vi "Execute Command.vi"(6 "Gantry In":refnum<class "Gantry.lvclass">, 7 "Console Log In":refnum<class "Console Log.lvclass">, 8 "error in (no error)":errorcluster, 9 "Pause in":bool, 10 "Command":string, 11 "gScript Interpreter in":refnum<class "gScript Interpreter.lvclass">) -> (0 "error out":errorcluster, 1 "Pause out":bool, 2 "End out":bool, 3 "gScript Interpreter out":refnum<class "gScript Interpreter.lvclass">, 4 "Gantry Out":refnum<class "Gantry.lvclass">, 5 "Console Log Out":refnum<class "Console Log.lvclass">)   [LabVIEW 2017, in "gScript Interpreter.lvclass"]
uses:
  gScript Interpreter.lvclass
  Shared Components/Gantry Class/Gantry.lvclass
  Application Utilities/Console Log/Console Log.lvclass
  gScript Interpreter.lvclass/gScript Interpreter.ctl
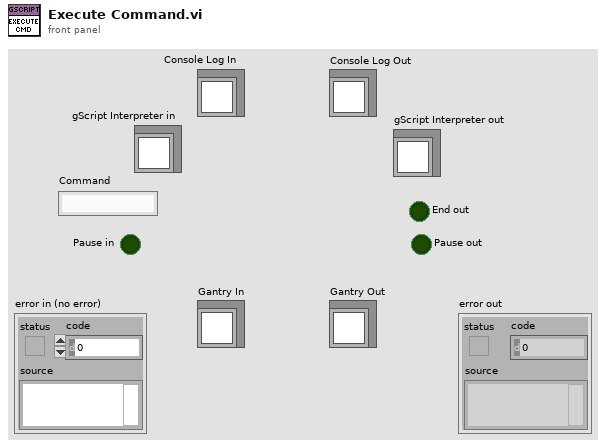
[diagram p1: front panel]
types:
  T1 = typedef "Command.ctl" = enum16{"", "PASS", "COPY", "PRINT", "GOTO", "GOTOIF", "GOTOIFN", "ADD", "SUB", "INC", "DEC", "HOME", "MOVEREL", "MOVENAME", "MOVETO", "GETPOS", "ROTATE", "GETROT", "SETVAC", "GETVAC", "JOYSTICK", "LOADTOOL", "UNLOADTOOL", "POTLINE", "POTDOT", "AUTOFOCUS", "FINDFID", "FIT", "WAIT", "MPGON", "MPGOFF", "PAUSE", "SNAPSHOT", "SETLOG", "CLEARLOG", "VIDEO", "TRANSFORMG2L", "TRANSFORML2G", "CHOICEPOPUP", "SETLIGHT", "CALL", "END", "DUMPSTATE", "FLEXREAD", "FLEXWRITE", "SURVEY", "LOADCONFIG", "SETERRORMODE", "COMPOSE", "INVERT", "EULER2QUAT", "QUAT2EULER", "MUL", "ROTATETO", "VERSION", "SIN", "COS", "TAN", "ATAN2", "ABS", "POW", "ACKFAULT", "MOVESAFE", "LOADSTAMP", "APPLYSTAMP", "UNLOADSTAMP", "LOADWEIGHT", "APPLYWEIGHT", "UNLOADWEIGHT", "RETURN", "GETFLOATPOPUP", "GETINTPOPUP", "GETVECPOPUP"}
  T2 = typedef "Error Mode.ctl" = enum16{"default", "prompt", "setvar"}
  T3 = typedef "Memory Cell.ctl" = cluster{"type":T4, "x":dbl, "y":dbl, "z":dbl, "w":dbl}
  T4 = typedef "Memory Cell Type Enum.ctl" = enum16{"integer", "float", "vector", "rotation"}
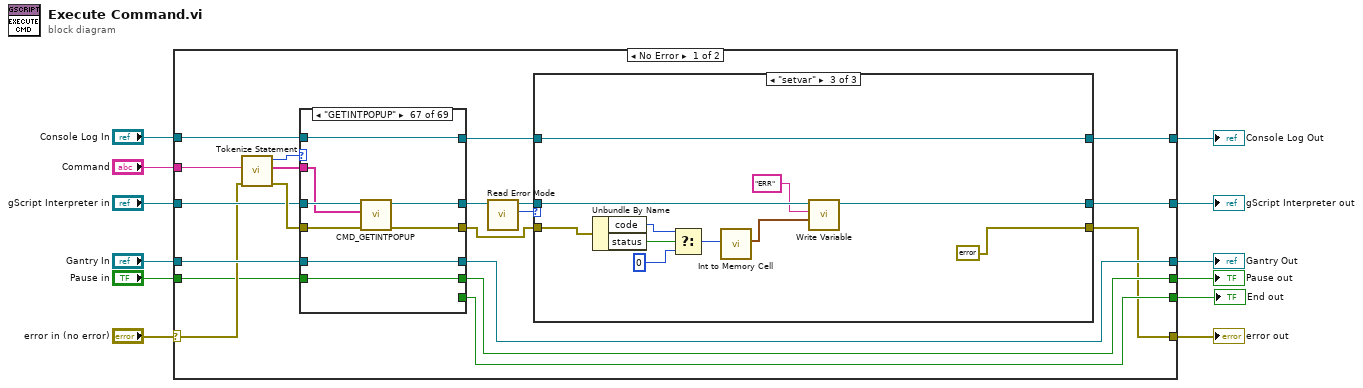
[diagram p0: block diagram]
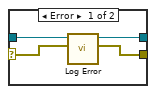
[diagram p3: hidden frame]
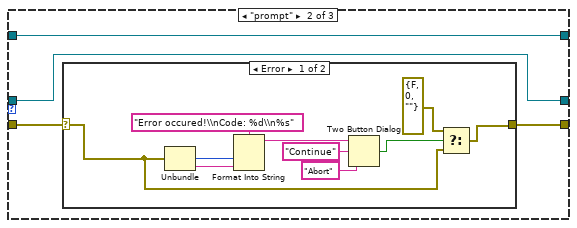
[diagram p4: hidden frame]
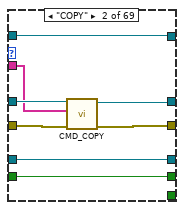
[diagram p7: hidden frame]
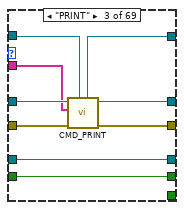
[diagram p8: hidden frame]
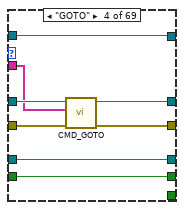
[diagram p9: hidden frame]
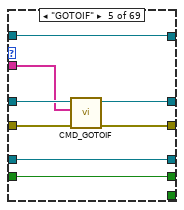
[diagram p10: hidden frame]
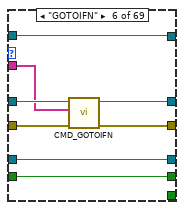
[diagram p11: hidden frame]
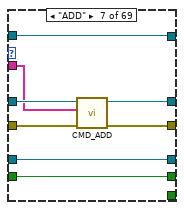
[diagram p12: hidden frame]
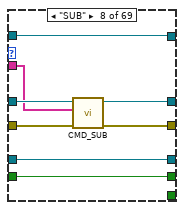
[diagram p13: hidden frame]
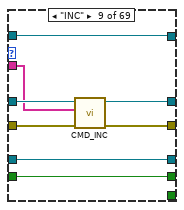
[diagram p14: hidden frame]
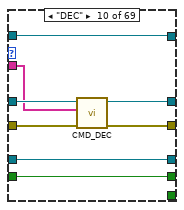
[diagram p15: hidden frame]
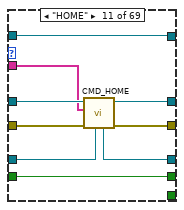
[diagram p16: hidden frame]
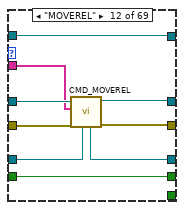
[diagram p17: hidden frame]
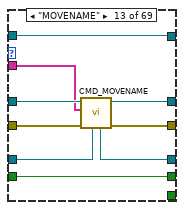
[diagram p18: hidden frame]
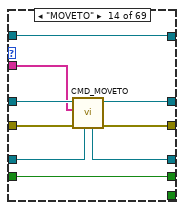
[diagram p19: hidden frame]
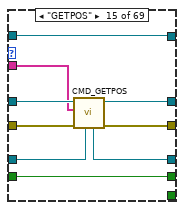
[diagram p20: hidden frame]
diagram:
  n1 = case shown="No Error" "error in (no error)" {
    selector: "error in (no error)" -> [w26 w662]
    tunnel: [w19 w662] -> w11
    tunnel: [w18 w661] -> w9
    tunnel: "gScript Interpreter in" -> [w28 w661]
    tunnel: "Gantry In" -> [w29 w659]
    tunnel: [w21 w659] -> w7
    tunnel: "Console Log In" -> [w27 w660]
    tunnel: [w16 w660] -> w5
    tunnel: "Pause in" -> [w25 w658]
    tunnel: [w22 w658] -> w3
    tunnel: "Command" -> [w24 _]
    tunnel: [w23 FALSE] -> w1
    frame No Error {
      n2 = call "Tokenize Statement.vi"("error in (no error)"=w26, "Command"=w24) -> ("error out"=w30:errorcluster, "Arguments"=w31:string[], "Command"=w32:T1)  [unwired: 5 in, 2 out]
      n3 = case shown="\"GETINTPOPUP\"" w32 {
        selector: w32 -> [_ _ _ _ _ _ _ _ _ _ _ _ _ _ _ _ _ _ _ _ _ _ _ _ _ _ _ _ _ _ _ _ _ _ _ _ _ _ _ _ _ _ _ _ _ _ _ _ _ _ _ _ _ _ _ _ _ _ _ _ _ w586 _ w605 w615 _ _ _ _]
        tunnel: w31 -> [_ w78 w87 w95 w102 w110 w118 w127 w135 w142 w150 w159 w172 w179 w186 w195 w204 w213 w222 w231 w244 w249 w263 w267 w276 w285 w294 w306 w311 w320 _ w339 w345 w351 w370 w376 w381 w389 w401 w409 _ w418 w429 w441 w453 w455 w464 w472 w480 w491 w499 w509 w512 w521 w529 w539 w545 w553 w564 w569 w581 w593 w596 w606 w617 w625 w633 w642 w649]
        tunnel: w30 -> [w72 w80 w89 w97 w104 w113 w121 w129 w137 w144 w155 w163 w171 w181 w190 w199 w208 w216 w224 w235 w243 w251 w262 w271 w280 w287 w298 w305 w313 w324 w330 w335 w344 w354 w365 w374 w380 w390 w400 w405 w412 w422 w433 w442 w447 w459 w466 w477 w484 w492 w500 w506 w518 w524 w534 w541 w548 w556 w565 w572 w580 w590 w600 w608 w621 w629 w636 w645 w652]
        tunnel: w28 -> [w74 w82 w91 w99 w107 w115 w123 w131 w139 w146 w156 w165 w174 w183 w192 w201 w210 w219 w228 w237 w246 w255 w264 w273 w282 w291 w300 w308 w317 w326 w331 w338 w347 w356 w369 w377 w385 w393 w402 w408 w415 w420 w435 w444 w452 w461 w468 w476 w486 w493 w502 w508 w519 w526 w535 w543 w551 w559 w567 w575 w583 w592 w599 w612 w623 w628 w639 w646 w654]
        tunnel: [w74 w81 w90 w98 w106 w114 w122 w130 w138 w145 w151 w164 w173 w182 w191 w200 w209 w214 w227 w236 w245 w254 w260 w272 w281 w290 w299 w307 w316 w325 w331 w337 w346 w355 w368 w375 w382 w392 w399 w407 w415 w419 w434 w443 w451 w460 w467 w475 w485 w490 w501 w507 w514 w525 w532 w542 w550 w558 w566 w574 w582 w591 w598 w611 w622 w627 w637 w641 w653] -> w20
        tunnel: [w72 w79 w88 w96 w103 w112 w120 w128 w136 w143 w154 w162 w168 w180 w189 w198 w207 w215 w223 w234 w242 w250 w261 w270 w279 w286 w297 w304 w312 w323 w330 w334 w343 w353 w364 w372 w379 w388 w398 w404 w412 w421 w432 w440 w446 w458 w465 w474 w483 w489 w498 w505 w515 w523 w533 w540 w547 w555 w563 w571 w579 w589 w597 w607 w620 w626 w634 w644 w651] -> w15
        tunnel: w29 -> [w73 w77 w86 w94 w105 w111 w119 w126 w134 w147 w153 w161 w170 w178 w188 w197 w206 w218 w226 w233 w241 w253 w259 w269 w278 w289 w296 w303 w315 w322 w329 w333 w342 w352 w367 w373 w384 w387 w397 w406 w414 w424 w431 w439 w449 w457 w469 w478 w482 w488 w497 w504 w517 w522 w530 w537 w546 w554 w561 w570 w578 w588 w602 w610 w619 w630 w635 w643 w650]
        tunnel: [w73 w77 w86 w94 w105 w111 w119 w126 w134 w147 w152 w160 w169 w177 w187 w196 w205 w217 w225 w232 w240 w252 w258 w268 w277 w288 w295 w303 w314 w321 w329 w332 w341 w352 w366 w373 w384 w387 w396 w406 w414 w423 w430 w438 w448 w456 w469 w478 w482 w488 w497 w504 w516 w522 w530 w537 w546 w554 w561 w570 w577 w587 w601 w609 w618 w630 w635 w643 w650] -> w21
        tunnel: w25 -> [w71 w76 w85 w93 w101 w109 w117 w125 w133 w141 w149 w158 w167 w176 w185 w194 w203 w212 w221 w230 w239 w248 w257 w266 w275 w284 w293 w302 w310 w319 _ w340 w350 w359 w362 w378 w386 w394 w403 w411 w417 w427 w436 w445 w454 w463 w471 w479 w487 w495 w503 w511 w520 w528 w536 w544 w552 w560 w568 w576 w585 w595 w604 w614 w624 w632 w640 w648 w656]
        tunnel: [w71 w76 w85 w93 w101 w109 w117 w125 w133 w141 w149 w158 w167 w176 w185 w194 w203 w212 w221 w230 w239 w248 w257 w266 w275 w284 w293 w302 w310 w319 TRUE w340 w350 w359 w360 w378 w386 w394 w403 w411 w417 w427 w436 w445 w454 w463 w471 w479 w487 w495 w503 w511 w520 w528 w536 w544 w552 w560 w568 w576 w585 w595 w604 w614 w624 w632 w640 w648 w656] -> w22
        tunnel: w27 -> [w70 w75 w84 w92 w100 w108 w116 w124 w132 w140 w148 w157 w166 w175 w184 w193 w202 w211 w220 w229 w238 w247 w256 w265 w274 w283 w292 w301 w309 w318 w327 w336 w349 w358 w363 w371 w383 w391 w395 w410 w416 w426 w428 w437 w450 w462 w470 w473 w481 w494 w496 w510 w513 w527 w531 w538 w549 w557 w562 w573 w584 w594 w603 w613 w616 w631 w638 w647 w655]
        tunnel: [w70 w75 w83 w92 w100 w108 w116 w124 w132 w140 w148 w157 w166 w175 w184 w193 w202 w211 w220 w229 w238 w247 w256 w265 w274 w283 w292 w301 w309 w318 w327 w336 w348 w357 w363 w371 w383 w391 w395 w410 w416 w425 w428 w437 w450 w462 w470 w473 w481 w494 w496 w510 w513 w527 w531 w538 w549 w557 w562 w573 w584 w594 w603 w613 w616 w631 w638 w647 w655] -> w17
        tunnel: [_ _ _ _ _ _ _ _ _ _ _ _ _ _ _ _ _ _ _ _ _ _ _ _ _ _ _ _ _ _ _ _ _ _ _ _ _ _ _ _ TRUE _ _ _ _ _ _ _ _ _ _ _ _ _ _ _ _ _ _ _ _ _ _ _ _ _ _ _ _] -> w23
        frame "PASS", Default {
        }
        frame "COPY" {
          n4 = call-dynamic "CMD_COPY.vi"("error in (no error)"=w80, "Arguments"=w78, "gScript Interpreter in"=w82) -> ("error out"=w79:errorcluster, "gScript Interpreter out"=w81:refnum<class "gScript Interpreter.lvclass">)  [unwired: 7 in]
        }
        frame "PRINT" {
          n5 = call-dynamic "CMD_PRINT.vi"("Console Log in"=w84, "error in (no error)"=w89, "Arguments"=w87, "gScript Interpreter in"=w91) -> ("error out"=w88:errorcluster, "gScript Interpreter out"=w90:refnum<class "gScript Interpreter.lvclass">, "Console Log out"=w83:refnum<class "Console Log.lvclass">)  [unwired: 5 in]
        }
        frame "GOTO" {
          n6 = call-dynamic "CMD_GOTO.vi"("error in (no error)"=w97, "Arguments"=w95, "gScript Interpreter in"=w99) -> ("error out"=w96:errorcluster, "gScript Interpreter out"=w98:refnum<class "gScript Interpreter.lvclass">)  [unwired: 7 in]
        }
        frame "GOTOIF" {
          n7 = call-dynamic "CMD_GOTOIF.vi"("error in (no error)"=w104, "Arguments"=w102, "gScript Interpreter in"=w107) -> ("error out"=w103:errorcluster, "gScript Interpreter out"=w106:refnum<class "gScript Interpreter.lvclass">)  [unwired: 7 in]
        }
        frame "GOTOIFN" {
          n8 = call-dynamic "CMD_GOTOIFN.vi"("error in (no error)"=w113, "Arguments"=w110, "gScript Interpreter in"=w115) -> ("error out"=w112:errorcluster, "gScript Interpreter out"=w114:refnum<class "gScript Interpreter.lvclass">)  [unwired: 7 in]
        }
        frame "ADD" {
          n9 = call-dynamic "CMD_ADD.vi"("error in (no error)"=w121, "Arguments"=w118, "gScript Interpreter in"=w123) -> ("error out"=w120:errorcluster, "gScript Interpreter out"=w122:refnum<class "gScript Interpreter.lvclass">)  [unwired: 7 in]
        }
        frame "SUB" {
          n10 = call-dynamic "CMD_SUB.vi"("error in (no error)"=w129, "Arguments"=w127, "gScript Interpreter in"=w131) -> ("error out"=w128:errorcluster, "gScript Interpreter out"=w130:refnum<class "gScript Interpreter.lvclass">)  [unwired: 7 in]
        }
        frame "INC" {
          n11 = call-dynamic "CMD_INC.vi"("error in (no error)"=w137, "Arguments"=w135, "gScript Interpreter in"=w139) -> ("error out"=w136:errorcluster, "gScript Interpreter out"=w138:refnum<class "gScript Interpreter.lvclass">)  [unwired: 7 in]
        }
        frame "DEC" {
          n12 = call-dynamic "CMD_DEC.vi"("error in (no error)"=w144, "Arguments"=w142, "gScript Interpreter in"=w146) -> ("error out"=w143:errorcluster, "gScript Interpreter out"=w145:refnum<class "gScript Interpreter.lvclass">)  [unwired: 7 in]
        }
        frame "HOME" {
          n13 = call-dynamic "CMD_HOME.vi"("Gantry in"=w153, "error in (no error)"=w155, "Arguments"=w150, "gScript Interpreter in"=w156) -> ("error out"=w154:errorcluster, "gScript Interpreter out"=w151:refnum<class "gScript Interpreter.lvclass">, "Gantry out"=w152:refnum<class "Gantry.lvclass">)  [unwired: 5 in]
        }
        frame "MOVEREL" {
          n14 = call-dynamic "CMD_MOVEREL.vi"("Gantry in"=w161, "error in (no error)"=w163, "Arguments"=w159, "gScript Interpreter in"=w165) -> ("error out"=w162:errorcluster, "gScript Interpreter out"=w164:refnum<class "gScript Interpreter.lvclass">, "Gantry out"=w160:refnum<class "Gantry.lvclass">)  [unwired: 5 in]
        }
        frame "MOVENAME" {
          n15 = call-dynamic "CMD_MOVENAME.vi"("Gantry in"=w170, "error in (no error)"=w171, "Arguments"=w172, "gScript Interpreter in"=w174) -> ("error out"=w168:errorcluster, "gScript Interpreter out"=w173:refnum<class "gScript Interpreter.lvclass">, "Gantry out"=w169:refnum<class "Gantry.lvclass">)  [unwired: 5 in]
        }
        frame "MOVETO" {
          n16 = call-dynamic "CMD_MOVETO.vi"("Gantry in"=w178, "error in (no error)"=w181, "Arguments"=w179, "gScript Interpreter in"=w183) -> ("error out"=w180:errorcluster, "gScript Interpreter out"=w182:refnum<class "gScript Interpreter.lvclass">, "Gantry out"=w177:refnum<class "Gantry.lvclass">)  [unwired: 5 in]
        }
        frame "GETPOS" {
          n17 = call-dynamic "CMD_GETPOS.vi"("Gantry in"=w188, "error in (no error)"=w190, "Arguments"=w186, "gScript Interpreter in"=w192) -> ("error out"=w189:errorcluster, "gScript Interpreter out"=w191:refnum<class "gScript Interpreter.lvclass">, "Gantry out"=w187:refnum<class "Gantry.lvclass">)  [unwired: 5 in]
        }
        frame "ROTATE" {
          n18 = call-dynamic "CMD_ROTATE.vi"("Gantry in"=w197, "error in (no error)"=w199, "Arguments"=w195, "gScript Interpreter in"=w201) -> ("error out"=w198:errorcluster, "gScript Interpreter out"=w200:refnum<class "gScript Interpreter.lvclass">, "Gantry out"=w196:refnum<class "Gantry.lvclass">)  [unwired: 5 in]
        }
        frame "GETROT" {
          n19 = call-dynamic "CMD_GETROT.vi"("Gantry in"=w206, "error in (no error)"=w208, "Arguments"=w204, "gScript Interpreter in"=w210) -> ("error out"=w207:errorcluster, "gScript Interpreter out"=w209:refnum<class "gScript Interpreter.lvclass">, "Gantry out"=w205:refnum<class "Gantry.lvclass">)  [unwired: 5 in]
        }
        frame "SETVAC" {
          n20 = call-dynamic "CMD_SETVAC.vi"("Gantry in"=w218, "error in (no error)"=w216, "Arguments"=w213, "gScript Interpreter in"=w219) -> ("error out"=w215:errorcluster, "gScript Interpreter out"=w214:refnum<class "gScript Interpreter.lvclass">, "Gantry out"=w217:refnum<class "Gantry.lvclass">)  [unwired: 5 in]
        }
        frame "GETVAC" {
          n21 = call-dynamic "CMD_GETVAC.vi"("Gantry in"=w226, "error in (no error)"=w224, "Arguments"=w222, "gScript Interpreter in"=w228) -> ("error out"=w223:errorcluster, "gScript Interpreter out"=w227:refnum<class "gScript Interpreter.lvclass">, "Gantry out"=w225:refnum<class "Gantry.lvclass">)  [unwired: 5 in]
        }
        frame "JOYSTICK" {
          n22 = call-dynamic "CMD_JOYSTICK.vi"("Gantry in"=w233, "error in (no error)"=w235, "Arguments"=w231, "gScript Interpreter in"=w237) -> ("error out"=w234:errorcluster, "gScript Interpreter out"=w236:refnum<class "gScript Interpreter.lvclass">, "Gantry out"=w232:refnum<class "Gantry.lvclass">)  [unwired: 5 in]
        }
        frame "LOADTOOL" {
          n23 = call-dynamic "CMD_LOADTOOL.vi"("Gantry in"=w241, "error in (no error)"=w243, "Arguments"=w244, "gScript Interpreter in"=w246) -> ("error out"=w242:errorcluster, "gScript Interpreter out"=w245:refnum<class "gScript Interpreter.lvclass">, "Gantry out"=w240:refnum<class "Gantry.lvclass">)  [unwired: 5 in]
        }
        frame "UNLOADTOOL" {
          n24 = call-dynamic "CMD_UNLOADTOOL.vi"("Gantry in"=w253, "error in (no error)"=w251, "Arguments"=w249, "gScript Interpreter in"=w255) -> ("error out"=w250:errorcluster, "gScript Interpreter out"=w254:refnum<class "gScript Interpreter.lvclass">, "Gantry out"=w252:refnum<class "Gantry.lvclass">)  [unwired: 5 in]
        }
        frame "POTLINE" {
          n25 = call-dynamic "CMD_POTLINE.vi"("Gantry in"=w259, "error in (no error)"=w262, "Arguments"=w263, "gScript Interpreter in"=w264) -> ("error out"=w261:errorcluster, "gScript Interpreter out"=w260:refnum<class "gScript Interpreter.lvclass">, "Gantry out"=w258:refnum<class "Gantry.lvclass">)  [unwired: 5 in]
        }
        frame "POTDOT" {
          n26 = call-dynamic "CMD_POTDOT.vi"("Gantry in"=w269, "error in (no error)"=w271, "Arguments"=w267, "gScript Interpreter in"=w273) -> ("error out"=w270:errorcluster, "gScript Interpreter out"=w272:refnum<class "gScript Interpreter.lvclass">, "Gantry out"=w268:refnum<class "Gantry.lvclass">)  [unwired: 5 in]
        }
        frame "AUTOFOCUS" {
          n27 = call-dynamic "CMD_AUTOFOCUS.vi"("Gantry in"=w278, "error in (no error)"=w280, "Arguments"=w276, "gScript Interpreter in"=w282) -> ("error out"=w279:errorcluster, "gScript Interpreter out"=w281:refnum<class "gScript Interpreter.lvclass">, "Gantry out"=w277:refnum<class "Gantry.lvclass">)  [unwired: 5 in]
        }
        frame "FINDFID" {
          n28 = call-dynamic "CMD_FINDFID.vi"("Gantry in"=w289, "error in (no error)"=w287, "Arguments"=w285, "gScript Interpreter in"=w291) -> ("error out"=w286:errorcluster, "gScript Interpreter out"=w290:refnum<class "gScript Interpreter.lvclass">, "Gantry out"=w288:refnum<class "Gantry.lvclass">)  [unwired: 5 in]
        }
        frame "FIT" {
          n29 = call-dynamic "CMD_FIT.vi"("Gantry in"=w296, "error in (no error)"=w298, "Arguments"=w294, "gScript Interpreter in"=w300) -> ("error out"=w297:errorcluster, "gScript Interpreter out"=w299:refnum<class "gScript Interpreter.lvclass">, "Gantry out"=w295:refnum<class "Gantry.lvclass">)  [unwired: 5 in]
        }
        frame "WAIT" {
          n30 = call-dynamic "CMD_WAIT.vi"("error in (no error)"=w305, "Arguments"=w306, "gScript Interpreter in"=w308) -> ("error out"=w304:errorcluster, "gScript Interpreter out"=w307:refnum<class "gScript Interpreter.lvclass">)  [unwired: 7 in]
        }
        frame "MPGON" {
          n31 = call-dynamic "CMD_MPGON.vi"("Gantry in"=w315, "error in (no error)"=w313, "Arguments"=w311, "gScript Interpreter in"=w317) -> ("error out"=w312:errorcluster, "gScript Interpreter out"=w316:refnum<class "gScript Interpreter.lvclass">, "Gantry out"=w314:refnum<class "Gantry.lvclass">)  [unwired: 5 in]
        }
        frame "MPGOFF" {
          n32 = call-dynamic "CMD_MPGOFF.vi"("Gantry in"=w322, "error in (no error)"=w324, "Arguments"=w320, "gScript Interpreter in"=w326) -> ("error out"=w323:errorcluster, "gScript Interpreter out"=w325:refnum<class "gScript Interpreter.lvclass">, "Gantry out"=w321:refnum<class "Gantry.lvclass">)  [unwired: 5 in]
        }
        frame "PAUSE" {
        }
        frame "SNAPSHOT" {
          n33 = call-dynamic "CMD_SNAPSHOT.vi"("Gantry in"=w333, "error in (no error)"=w335, "Arguments"=w339, "gScript Interpreter in"=w338) -> ("error out"=w334:errorcluster, "gScript Interpreter out"=w337:refnum<class "gScript Interpreter.lvclass">, "Gantry out"=w332:refnum<class "Gantry.lvclass">)  [unwired: 5 in]
        }
        frame "SETLOG" {
          n34 = call-dynamic "CMD_SETLOG.vi"("Gantry Class in"=w342, "Console Log in"=w349, "error in (no error)"=w344, "Arguments"=w345, "gScript Interpreter in"=w347) -> ("error out"=w343:errorcluster, "gScript Interpreter out"=w346:refnum<class "gScript Interpreter.lvclass">, "Gantry Class out"=w341:refnum<class "Gantry.lvclass">, "Console Log out"=w348:refnum<class "Console Log.lvclass">)  [unwired: 3 in]
        }
        frame "CLEARLOG" {
          n35 = call-dynamic "CMD_CLEARLOG.vi"("Console Log in"=w358, "error in (no error)"=w354, "Arguments"=w351, "gScript Interpreter in"=w356) -> ("error out"=w353:errorcluster, "gScript Interpreter out"=w355:refnum<class "gScript Interpreter.lvclass">, "Console Log out"=w357:refnum<class "Console Log.lvclass">)  [unwired: 5 in]
        }
        frame "VIDEO" {
          n36 = call-dynamic "CMD_VIDEO.vi"("Gantry in"=w367, "error in (no error)"=w365, "Arguments"=w370, "gScript Interpreter in"=w369) -> ("error out"=w364:errorcluster, "Pause out"=w361:bool, "gScript Interpreter out"=w368:refnum<class "gScript Interpreter.lvclass">, "Gantry out"=w366:refnum<class "Gantry.lvclass">)  [unwired: 4 in]
          n37 = Or(x=w361, y=w362) -> (x .or. y?=w360:bool)
        }
        frame "TRANSFORMG2L" {
          n38 = call-dynamic "CMD_TRANSFORMG2L.vi"("error in (no error)"=w374, "Arguments"=w376, "gScript Interpreter in"=w377) -> ("error out"=w372:errorcluster, "gScript Interpreter out"=w375:refnum<class "gScript Interpreter.lvclass">)  [unwired: 7 in]
        }
        frame "TRANSFORML2G" {
          n39 = call-dynamic "CMD_TRANSFORML2G.vi"("error in (no error)"=w380, "Arguments"=w381, "gScript Interpreter in"=w385) -> ("error out"=w379:errorcluster, "gScript Interpreter out"=w382:refnum<class "gScript Interpreter.lvclass">)  [unwired: 7 in]
        }
        frame "CHOICEPOPUP" {
          n40 = call-dynamic "CMD_CHOICEPOPUP.vi"("error in (no error)"=w390, "Arguments"=w389, "gScript Interpreter in"=w393) -> ("error out"=w388:errorcluster, "gScript Interpreter out"=w392:refnum<class "gScript Interpreter.lvclass">)  [unwired: 7 in]
        }
        frame "SETLIGHT" {
          n41 = call-dynamic "CMD_SETLIGHT.vi"("Gantry in"=w397, "error in (no error)"=w400, "Arguments"=w401, "gScript Interpreter in"=w402) -> ("error out"=w398:errorcluster, "gScript Interpreter out"=w399:refnum<class "gScript Interpreter.lvclass">, "Gantry out"=w396:refnum<class "Gantry.lvclass">)  [unwired: 5 in]
        }
        frame "CALL" {
          n42 = call-dynamic "CMD_CALL.vi"("error in (no error)"=w405, "Arguments"=w409, "gScript Interpreter in"=w408) -> ("error out"=w404:errorcluster, "gScript Interpreter out"=w407:refnum<class "gScript Interpreter.lvclass">)  [unwired: 7 in]
        }
        frame "END" {
        }
        frame "DUMPSTATE" {
          n43 = call-dynamic "CMD_DUMPSTATE.vi"("Gantry in"=w424, "Console Log in"=w426, "error in (no error)"=w422, "Arguments"=w418, "gScript Interpreter in"=w420) -> ("error out"=w421:errorcluster, "gScript Interpreter out"=w419:refnum<class "gScript Interpreter.lvclass">, "Gantry out"=w423:refnum<class "Gantry.lvclass">, "Console Log out"=w425:refnum<class "Console Log.lvclass">)  [unwired: 3 in]
        }
        frame "FLEXREAD" {
          n44 = call-dynamic "CMD_FLEXREAD.vi"("Gantry Class in"=w431, "error in (no error)"=w433, "Arguments"=w429, "gScript Interpreter in"=w435) -> ("error out"=w432:errorcluster, "gScript Interpreter out"=w434:refnum<class "gScript Interpreter.lvclass">, "Gantry Class out"=w430:refnum<class "Gantry.lvclass">)  [unwired: 5 in]
        }
        frame "FLEXWRITE" {
          n45 = call-dynamic "CMD_FLEXWRITE.vi"("Gantry Class in"=w439, "error in (no error)"=w442, "Arguments"=w441, "gScript Interpreter in"=w444) -> ("error out"=w440:errorcluster, "gScript Interpreter out"=w443:refnum<class "gScript Interpreter.lvclass">, "Gantry Class out"=w438:refnum<class "Gantry.lvclass">)  [unwired: 5 in]
        }
        frame "SURVEY" {
          n46 = call-dynamic "CMD_SURVEY.vi"("Gantry in"=w449, "error in (no error)"=w447, "Arguments"=w453, "gScript Interpreter in"=w452) -> ("error out"=w446:errorcluster, "gScript Interpreter out"=w451:refnum<class "gScript Interpreter.lvclass">, "Gantry out"=w448:refnum<class "Gantry.lvclass">)  [unwired: 5 in]
        }
        frame "LOADCONFIG" {
          n47 = call-dynamic "CMD_LOADCONFIG.vi"("Gantry Class in"=w457, "error in (no error)"=w459, "Arguments"=w455, "gScript Interpreter in"=w461) -> ("error out"=w458:errorcluster, "gScript Interpreter out"=w460:refnum<class "gScript Interpreter.lvclass">, "Gantry Class out"=w456:refnum<class "Gantry.lvclass">)  [unwired: 5 in]
        }
        frame "SETERRORMODE" {
          n48 = call-dynamic "CMD_SETERRORMODE.vi"("error in (no error)"=w466, "Arguments"=w464, "gScript Interpreter in"=w468) -> ("error out"=w465:errorcluster, "gScript Interpreter out"=w467:refnum<class "gScript Interpreter.lvclass">)  [unwired: 7 in]
        }
        frame "COMPOSE" {
          n49 = call-dynamic "CMD_COMPOSE.vi"("error in (no error)"=w477, "Arguments"=w472, "gScript Interpreter in"=w476) -> ("error out"=w474:errorcluster, "gScript Interpreter out"=w475:refnum<class "gScript Interpreter.lvclass">)  [unwired: 7 in]
        }
        frame "INVERT" {
          n50 = call-dynamic "CMD_INVERT.vi"("error in (no error)"=w484, "Arguments"=w480, "gScript Interpreter in"=w486) -> ("error out"=w483:errorcluster, "gScript Interpreter out"=w485:refnum<class "gScript Interpreter.lvclass">)  [unwired: 7 in]
        }
        frame "EULER2QUAT" {
          n51 = call-dynamic "CMD_EULER2QUAT.vi"("error in (no error)"=w492, "Arguments"=w491, "gScript Interpreter in"=w493) -> ("error out"=w489:errorcluster, "gScript Interpreter out"=w490:refnum<class "gScript Interpreter.lvclass">)  [unwired: 7 in]
        }
        frame "QUAT2EULER" {
          n52 = call-dynamic "CMD_QUAT2EULER.vi"("error in (no error)"=w500, "Arguments"=w499, "gScript Interpreter in"=w502) -> ("error out"=w498:errorcluster, "gScript Interpreter out"=w501:refnum<class "gScript Interpreter.lvclass">)  [unwired: 7 in]
        }
        frame "MUL" {
          n53 = call-dynamic "CMD_MUL.vi"("error in (no error)"=w506, "Arguments"=w509, "gScript Interpreter in"=w508) -> ("error out"=w505:errorcluster, "gScript Interpreter out"=w507:refnum<class "gScript Interpreter.lvclass">)  [unwired: 7 in]
        }
        frame "ROTATETO" {
          n54 = call-dynamic "CMD_ROTATETO.vi"("Gantry in"=w517, "error in (no error)"=w518, "Arguments"=w512, "gScript Interpreter in"=w519) -> ("error out"=w515:errorcluster, "gScript Interpreter out"=w514:refnum<class "gScript Interpreter.lvclass">, "Gantry out"=w516:refnum<class "Gantry.lvclass">)  [unwired: 5 in]
        }
        frame "VERSION" {
          n55 = call-dynamic "CMD_VERSION.vi"("error in (no error)"=w524, "Arguments"=w521, "gScript Interpreter in"=w526) -> ("error out"=w523:errorcluster, "gScript Interpreter out"=w525:refnum<class "gScript Interpreter.lvclass">)  [unwired: 7 in]
        }
        frame "SIN" {
          n56 = call-dynamic "CMD_SIN.vi"("error in (no error)"=w534, "Arguments"=w529, "gScript Interpreter in"=w535) -> ("error out"=w533:errorcluster, "gScript Interpreter out"=w532:refnum<class "gScript Interpreter.lvclass">)  [unwired: 7 in]
        }
        frame "COS" {
          n57 = call-dynamic "CMD_COS.vi"("error in (no error)"=w541, "Arguments"=w539, "gScript Interpreter in"=w543) -> ("error out"=w540:errorcluster, "gScript Interpreter out"=w542:refnum<class "gScript Interpreter.lvclass">)  [unwired: 7 in]
        }
        frame "TAN" {
          n58 = call-dynamic "CMD_TAN.vi"("error in (no error)"=w548, "Arguments"=w545, "gScript Interpreter in"=w551) -> ("error out"=w547:errorcluster, "gScript Interpreter out"=w550:refnum<class "gScript Interpreter.lvclass">)  [unwired: 7 in]
        }
        frame "ATAN2" {
          n59 = call-dynamic "CMD_ATAN2.vi"("error in (no error)"=w556, "Arguments"=w553, "gScript Interpreter in"=w559) -> ("error out"=w555:errorcluster, "gScript Interpreter out"=w558:refnum<class "gScript Interpreter.lvclass">)  [unwired: 7 in]
        }
        frame "ABS" {
          n60 = call-dynamic "CMD_ABS.vi"("error in (no error)"=w565, "Arguments"=w564, "gScript Interpreter in"=w567) -> ("error out"=w563:errorcluster, "gScript Interpreter out"=w566:refnum<class "gScript Interpreter.lvclass">)  [unwired: 7 in]
        }
        frame "POW" {
          n61 = call-dynamic "CMD_POW.vi"("error in (no error)"=w572, "Arguments"=w569, "gScript Interpreter in"=w575) -> ("error out"=w571:errorcluster, "gScript Interpreter out"=w574:refnum<class "gScript Interpreter.lvclass">)  [unwired: 7 in]
        }
        frame "ACKFAULT" {
          n62 = call-dynamic "CMD_ACKFAULT.vi"("Gantry in"=w578, "error in (no error)"=w580, "Arguments"=w581, "gScript Interpreter in"=w583) -> ("error out"=w579:errorcluster, "gScript Interpreter out"=w582:refnum<class "gScript Interpreter.lvclass">, "Gantry out"=w577:refnum<class "Gantry.lvclass">)  [unwired: 5 in]
        }
        frame "LOADSTAMP", "LOADWEIGHT" {
          n63 = call-dynamic "CMD_LOADSTAMP.vi"("Gantry in"=w588, "error in (no error)"=w590, "Command"=w586, "Arguments"=w593, "gScript Interpreter in"=w592) -> ("error out"=w589:errorcluster, "gScript Interpreter out"=w591:refnum<class "gScript Interpreter.lvclass">, "Gantry out"=w587:refnum<class "Gantry.lvclass">)  [unwired: 4 in]
        }
        frame "MOVESAFE" {
          n64 = call-dynamic "CMD_MOVESAFE.vi"("Gantry in"=w602, "error in (no error)"=w600, "Arguments"=w596, "gScript Interpreter in"=w599) -> ("error out"=w597:errorcluster, "gScript Interpreter out"=w598:refnum<class "gScript Interpreter.lvclass">, "Gantry out"=w601:refnum<class "Gantry.lvclass">)  [unwired: 5 in]
        }
        frame "UNLOADSTAMP", "UNLOADWEIGHT" {
          n65 = call "CMD_UNLOADSTAMP.vi"("Gantry in"=w610, "error in (no error)"=w608, "Command"=w605, "Arguments"=w606, "gScript Interpreter in"=w612) -> ("error out"=w607:errorcluster, "gScript Interpreter out"=w611:refnum<class "gScript Interpreter.lvclass">, "Gantry out"=w609:refnum<class "Gantry.lvclass">)  [unwired: 4 in]
        }
        frame "APPLYSTAMP", "APPLYWEIGHT" {
          n66 = call "CMD_APPLYSTAMP.vi"("Gantry in"=w619, "error in (no error)"=w621, "Command"=w615, "Arguments"=w617, "gScript Interpreter in"=w623) -> ("error out"=w620:errorcluster, "gScript Interpreter out"=w622:refnum<class "gScript Interpreter.lvclass">, "Gantry out"=w618:refnum<class "Gantry.lvclass">)  [unwired: 4 in]
        }
        frame "RETURN" {
          n67 = call-dynamic "CMD_RETURN.vi"("error in (no error)"=w629, "Arguments"=w625, "gScript Interpreter in"=w628) -> ("error out"=w626:errorcluster, "gScript Interpreter out"=w627:refnum<class "gScript Interpreter.lvclass">)  [unwired: 7 in]
        }
        frame "GETINTPOPUP" {
          n68 = call-dynamic "CMD_GETINTPOPUP.vi"("error in (no error)"=w636, "Arguments"=w633, "gScript Interpreter in"=w639) -> ("error out"=w634:errorcluster, "gScript Interpreter out"=w637:refnum<class "gScript Interpreter.lvclass">)  [unwired: 7 in]
        }
        frame "GETVECPOPUP" {
          n69 = call-dynamic "CMD_GETVECPOPUP.vi"("error in (no error)"=w645, "Arguments"=w642, "gScript Interpreter in"=w646) -> ("error out"=w644:errorcluster, "gScript Interpreter out"=w641:refnum<class "gScript Interpreter.lvclass">)  [unwired: 7 in]
        }
        frame "GETFLOATPOPUP" {
          n70 = call-dynamic "CMD_GETFLOATPOPUP.vi"("error in (no error)"=w652, "Arguments"=w649, "gScript Interpreter in"=w654) -> ("error out"=w651:errorcluster, "gScript Interpreter out"=w653:refnum<class "gScript Interpreter.lvclass">)  [unwired: 7 in]
        }
      }
      n71 = call "Read Error Mode.vi"("gScript Interpreter in"=w20) -> ("Error Mode"=w13:T2, "gScript Interpreter out"=w14:refnum<class "gScript Interpreter.lvclass">)  [unwired: 8 in, 1 out]
      n72 = case shown="\"setvar\"" w13 {
        tunnel: w15 -> [w33 w45 w64]
        tunnel: w14 -> [w37 w44 w69]
        tunnel: [w34 w47 errorcluster {"status"=FALSE, "code"=0, "source"=""} ("error constant")] -> w19
        tunnel: [w37 w44 w66] -> w18
        tunnel: w17 -> [w36 w46 w68]
        tunnel: [w35 w46 w68] -> w16
        frame "default", Default {
          n73 = case shown="No Error" w33 {
            selector: w33 -> [w38 w42]
            tunnel: w36 -> [w41 w43]
            tunnel: [w40 w43] -> w35
            tunnel: [w39 w42] -> w34
            frame Error {
              n74 = call "Log Error.vi"("error in"=w38, "Console Log in"=w41) -> ("error out"=w39:errorcluster, "Console Log out"=w40:refnum<class "Console Log.lvclass">)  [unwired: 8 in]
            }
            frame No Error {
            }
          }
        }
        frame "prompt" {
          n75 = case shown="Error" w45 {
            selector: w45 -> [w48 w58]
            tunnel: [w50 w58] -> w47
            frame Error {
              n76 = Unbundle(w48) -> ("code"=w57:i32, "source"=w56:string)  [unwired: 1 out]
              n77 = Format Into String(format string="Error occured!\\nCode: %d\\n%s", w57, w56) -> (resulting string=w55:string)  [unwired: 2 in, 1 out]
              n78 = Two Button Dialog(message=w55, 1:"Abort" ("F button name (\"Cancel\")"), 2:"Continue" ("T button name (\"OK\")")) -> (T button?=w52:bool)
              n79 = Select(t=errorcluster {"status"=FALSE, "code"=0, "source"=""}, s=w52, f=w48) -> (s? t:f=w50:errorcluster)
            }
            frame No Error {
            }
          }
        }
        frame "setvar" {
          n80 = Unbundle By Name(w64) -> ("code"=w59:i32, "status"=w63:bool)
          n81 = Select(t=w59, s=w63, f=0) -> (s? t:f=w61:i32)
          n82 = call "Int to Memory Cell.vi"("Numeric"=w61) -> ("Memory Cell"=w60:T3)  [unwired: 10 in]
          n83 = call-dynamic "Write Variable.vi"("Memory Cell"=w60, "Variable Name"="ERR", "gScript Interpreter in"=w69) -> ("gScript Interpreter out"=w66:refnum<class "gScript Interpreter.lvclass">)  [unwired: 7 in, 1 out]
        }
      }
    }
    frame Error {
    }
  }
  "error out" <- w11
  "gScript Interpreter out" <- w9
  "Gantry Out" <- w7
  "Console Log Out" <- w5
  "Pause out" <- w3
  "End out" <- w1
